vi "drawTempRectangle.vi"(0 "reference":refnum<class "Graphics.lvclass">, 1 "rectangle":T1 {"height" format="%.2f"; "width" format="%.2f"; "y" format="%.2f"; "x" format="%.2f"}, 2 "lineWidth(1)":dbl=1.0 format="%.2f", 3 "color(if not used=default color)":u32=33554432 format="%.0x", 4 "fill?(F)":bool, 5 "error in (no error)":errorcluster, 6 "Rectangles":T1[](array[typedef]) {"height" format="%.2f"; "width" format="%.2f"; "y" format="%.2f"; "x" format="%.2f"}, 7 "readFromMaster(True)":bool=TRUE) -> (14 "reference out":refnum<class "Graphics.lvclass">, 19 "error out":errorcluster)   [LabVIEW 2014, in "Graphics.lvclass"]
doc: "Draws a rectangle"
uses:
  <resource>/Framework/Providers/Open_GDS/UML/Graphics_class/Graphics.lvclass
  <resource>/Framework/Providers/Open_GDS/UML/General/Rectangle/Rectangle Rectangle2D.ctl
panel:
  # "Always set\nVI Server class\nto current VI. Do not\nconnect this control\nto the connector pane.\n(Tip!: Just drag\nand drop the icon\ninto the refnum)"
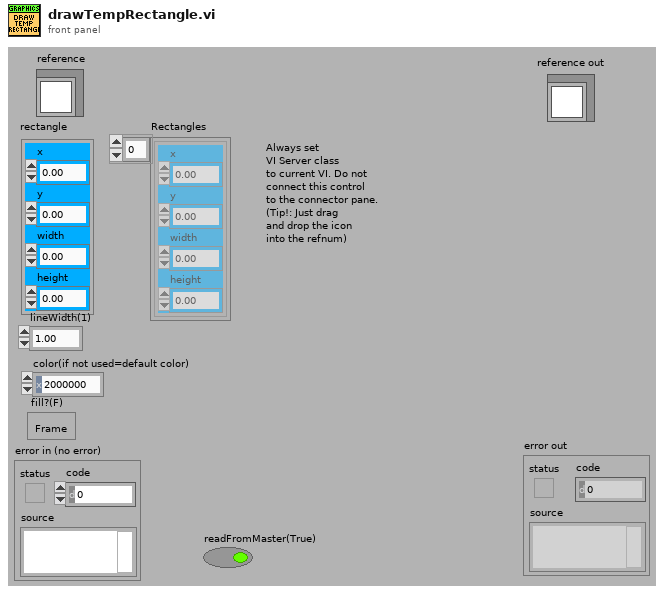
[diagram p1: front panel]
types:
  T1 = typedef "Rectangle Rectangle2D.ctl" = cluster{"x":dbl, "y":dbl, "width":dbl, "height":dbl}
  T2 = typedef "Graphics.lvclass/ObjectAttributes.ctl" = cluster{"drawColor":u32, "backgroundColor":u32, "font":T3, "fontType":T4, "picture":picture, "stroke":T5, "scaleX":dbl, "scaleY":dbl, "screenRef":refnum<vi>, "offsetX":dbl, "offsetY":dbl}
  T3 = typedef "Graphics.lvclass/FontType.ctl" = cluster{"Font Name:":string, "Size":i16, "Strikeout?":bool, "Italic?":bool, "Underline?":bool, "Outline?":bool, "Shadow?":bool, "Bold?":bool}
  T4 = typedef "Graphics.lvclass/LvFontType.ctl" = enum16{"User-specified Font", "Application Font", "System Font", "Dialog Font"}
  T5 = typedef "Graphics.lvclass/StrokeType.ctl" = enum16{"USE_DEFAULT", "SOLID", "DOTTED"}
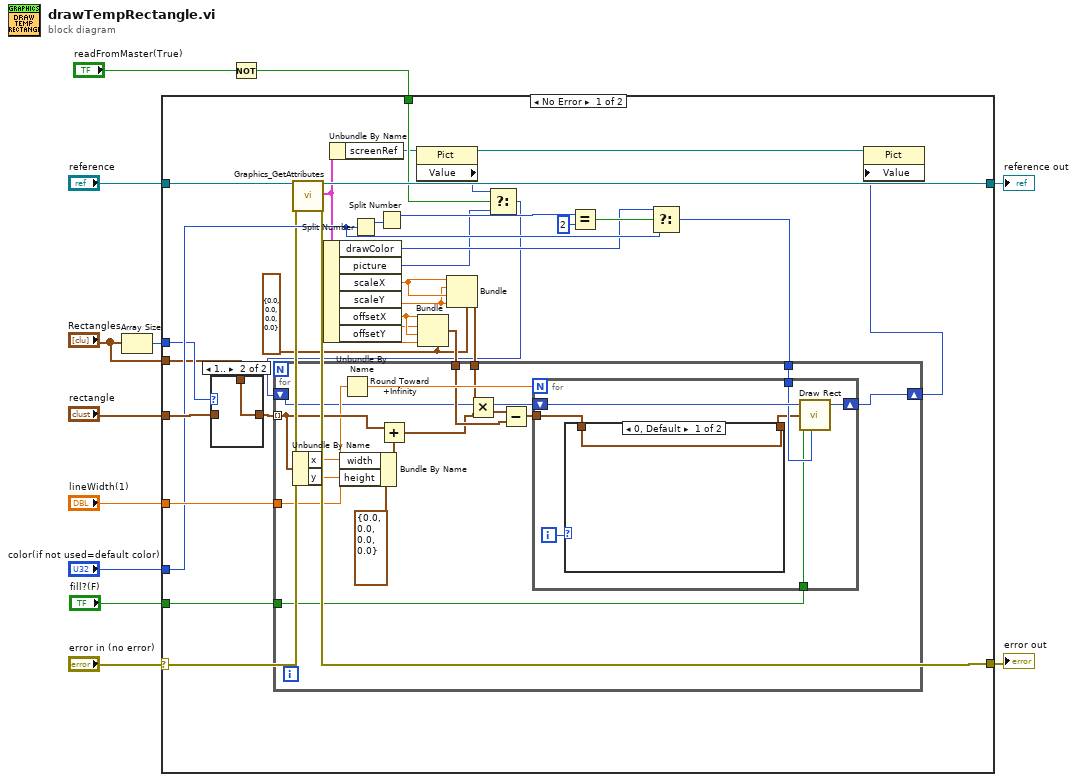
[diagram p0: block diagram]
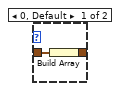
[diagram p2: hidden frame]
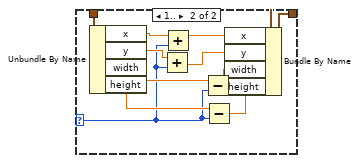
[diagram p3: hidden frame]
diagram:
  n1 = Array Size(array="Rectangles") -> (size(s)=w2:i32)
  n2 = Not(x="readFromMaster(True)") -> (.not. x?=w3:bool)
  n3 = case shown="No Error" "error in (no error)" {
    selector: "error in (no error)" -> [w35 w82]
    tunnel: "reference" -> [w43 w83]
    tunnel: [w42 w82] -> w11
    tunnel: [w41 w83] -> w10
    tunnel: "rectangle" -> [w40 _]
    tunnel: "lineWidth(1)" -> [w39 _]
    tunnel: "color(if not used=default color)" -> [w38 _]
    tunnel: "fill?(F)" -> [w37 _]
    tunnel: w3 -> [w36 _]
    tunnel: w2 -> [w16 _]
    tunnel: "Rectangles" -> [w15 _]
    frame No Error {
      w18 = T1 {"x"=0.0, "y"=0.0, "width"=0.0, "height"=0.0} ("rectangle")
      n4 = case shown="1.." w16 {
        tunnel: w40 -> [w45 _]
        tunnel: [w44 w46] -> w17
        tunnel: w15 -> [_ w46]
        frame 0, Default {
          n5 = Build Array(w45) -> (w44:T1[])
        }
        frame 1.. {
        }
      }
      n6 = call <resource>:"Graphics_GetAttributes.vi"("reference in"=w43, "error in (no error)"=w35) -> ("reference out"=w41:refnum<class "Graphics.lvclass">, "Data"=w13:T2, "error out"=w42:errorcluster)  [unwired: 1 in, 14 out]
      n7 = Unbundle By Name(w13) -> ("drawColor"=w30:u32, "picture"=w20:picture, "scaleX"=w27:dbl, "scaleY"=w26:dbl, "offsetX"=w25:dbl, "offsetY"=w24:dbl)
      n8 = Unbundle By Name(w13) -> ("screenRef"=w22:refnum<vi>)
      n9 = Split Number(x=w38) -> (hi(x)=w34:u16)  [unwired: 1 out]
      n10 = Split Number(x=w34) -> (hi(x)=w33:u8)  [unwired: 1 out]
      n11 = property class="Pict"(reference=w22) -> ("Value"=w21:picture)  [unwired: 1 in, 2 out]
      n12 = Bundle(cluster=w18, "x"=w25, "y"=w24, "width"=w25, "height"=w24) -> (w23:T1)
      n13 = Bundle(cluster=w18, "x"=w27, "y"=w26, "width"=w27, "height"=w26) -> (w28:T1)
      n14 = Select(t=w21, s=w36, f=w20) -> (s? t:f=w14:picture)
      n15 = Equal?(x=w33, y=u8 2) -> (x = y?=w31:bool)
      n16 = Select(t=w30, s=w31, f=w38) -> (s? t:f=w29:u32)
      n17 = for {
        tunnel: w17 -> [w62] mode=indexing
        tunnel: w39 -> [w61]
        tunnel: w37 -> [w60]
        tunnel: w29 -> [w58]
        tunnel: w28 -> [w57]
        tunnel: w23 -> [w50]
        shift-right: [w48] -> w19
        shift-left: w14 -> [w47]
        n18 = Unbundle By Name(w62) -> ("x"=w55:dbl, "y"=w54:dbl)
        n19 = Bundle By Name(cluster=T1 {"x"=0.0, "y"=0.0, "width"=0.0, "height"=0.0} ("x"), "width"=w55, "height"=w54) -> (w53:T1)
        n20 = Round Toward +Infinity(x=w61) -> (ceil(x): smallest int >= x=w59:dbl)
        n21 = Add(x=w62, y=w53) -> (x+y=w49:T1)
        n22 = Multiply(x=w57, y=w49) -> (x*y=w52:T1)
        n23 = Subtract(x=w52, y=w50) -> (x-y=w51:T1)
        n24 = for {
          N: w59 -> [_]
          tunnel: w51 -> [w65]
          tunnel: w58 -> [w68]
          shift-right: [w67] -> w48
          shift-left: w47 -> [w69]
          tunnel: w60 -> [w63]
          i -> [w64]
          n25 = case shown="0, Default" w64 {
            selector: w64 -> [_ w71]
            tunnel: [w70 w73] -> w66
            tunnel: w65 -> [w70 w72]
            frame 0, Default {
            }
            frame 1.. {
              n26 = Unbundle By Name(w72) -> ("x"=w81:dbl, "y"=w80:dbl, "width"=w79:dbl, "height"=w78:dbl)
              n27 = Add(x=w80, y=w71) -> (x+y=w76:dbl)
              n28 = Add(x=w81, y=w71) -> (x+y=w77:dbl)
              n29 = Subtract(x=w79, y=w71) -> (x-y=w75:dbl)
              n30 = Subtract(x=w78, y=w71) -> (x-y=w74:dbl)
              n31 = Bundle By Name(cluster=w72, "x"=w77, "y"=w76, "width"=w75, "height"=w74) -> (w73:T1)
            }
          }
          n32 = call <vilib>:"Draw Rect.vi"("picture"=w69, "rect"=w66, "fill?(F)"=w63, "color(black)"=w68) -> ("new picture"=w67:picture)  [unwired: 1 in, 4 out]
        }
      }
      n33 = property class="Pict"(reference=w22, "Value"=w19) -> ()  [unwired: 1 in, 2 out]
    }
    frame Error {
    }
  }
  "reference out" <- w10
  "error out" <- w11
